vi "Send Data to Multi DMM.vi"(8 "error in (no error)":errorcluster, 11 "BMC in":refnum<class "BMC.lvclass">) -> (0 "error out":errorcluster, 3 "BMC out":refnum<class "BMC.lvclass">)   [LabVIEW 2012, in "BMC.lvclass"]
uses:
  BMC.lvclass
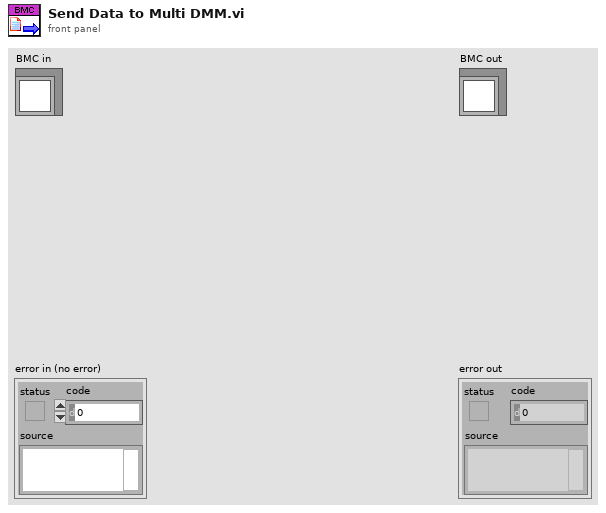
[diagram p1: front panel]
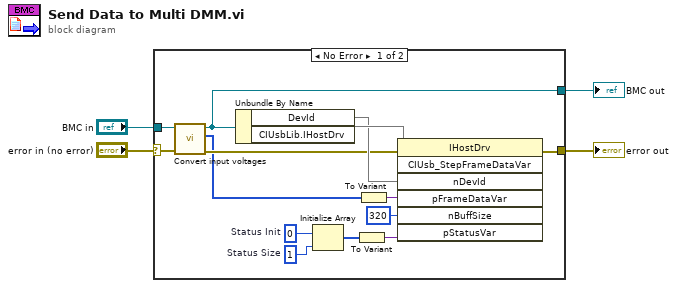
[diagram p0: block diagram]
diagram:
  n1 = case shown="No Error" "error in (no error)" {
    selector: "error in (no error)" -> [w9 w20]
    tunnel: [w12 w20] -> w3
    tunnel: [w5 w19] -> w1
    tunnel: "BMC in" -> [w6 w19]
    frame No Error {
      w16 = 1  # Status Size
      w15 = 0  # Status Init
      n2 = call-dynamic "Convert input voltages.vi"("error in (no error)"=w9, "BMC in"=w6) -> ("error out"=w8:errorcluster, "Command Array"=w7:i16[], "BMC out"=w5:refnum<class "BMC.lvclass">)  [unwired: 7 in]
      n3 = Unbundle By Name(w5) -> ("DevId"=w10, "CIUsbLib.IHostDrv"=w11)
      n4 = Initialize Array(w15, w16) -> (w14:i32[])
      n5 = To Variant(anything=w14) -> (Variant=w13:variant)
      n6 = To Variant(anything=w7) -> (Variant=w18:variant)
      n7 = invoke class="IHostDrv" method="CIUsb_StepFrameDataVar"(reference=w11, error in=w8, "nDevId"=w10, "pFrameDataVar"=w18, "nBuffSize"=320, "pStatusVar"=w13) -> (error out=w12:errorcluster)  [unwired: 1 in, 6 out]
    }
    frame Error {
    }
  }
  "error out" <- w3
  "BMC out" <- w1
